vi "Launcher.vi"(8 "error in (no error)":errorcluster, 11 "Launch Local?":bool) -> (0 "error out":errorcluster)   [LabVIEW 2026, in "TALOS.lvlib"]
uses:
  TALOS.lvlib
  Guardian/Guardian/Guardian.lvclass
  C:/LabVIEW Code/TALOS/talos/Ancestor/Ancestor/Ancestor.lvclass
  C:/LabVIEW Code/TALOS/builds/Actor Framework PPL/Actor Framework.lvlibp/1abvi3w/vi.lib/ActorFramework/Actor/Actor.lvclass
  Ancestor/Ancestor/Ancestor.lvclass/Ancestor.ctl
  Support VIs/Global Constants.vi
  Support VIs/Global Memory.vi
  builds/Actor Framework PPL/Actor Framework.lvlibp/1abvi3w/vi.lib/ActorFramework/Actor/Actor.lvclass
  Ancestor/Ancestor/Ancestor.lvclass
panel:
  # "This is just the launcher VI: it only bootstrap the Guardian of this project."
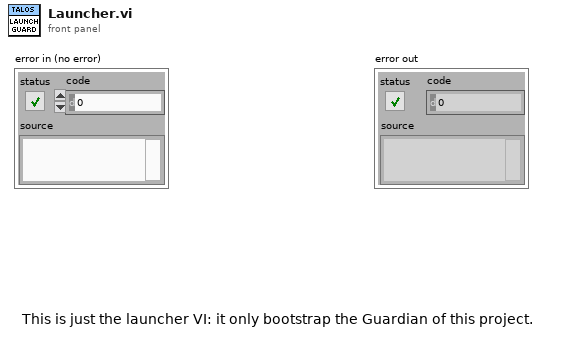
[diagram p1: front panel]
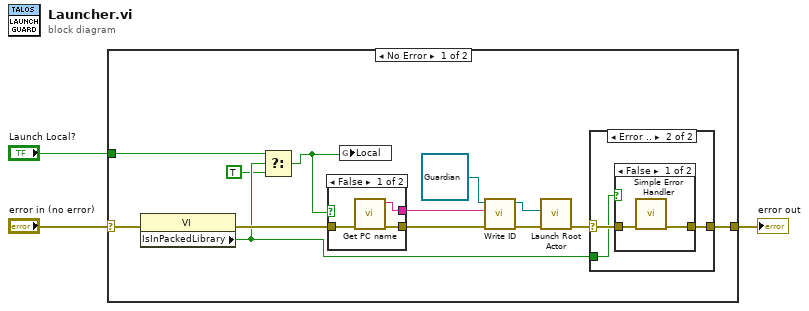
[diagram p0: block diagram]
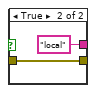
[diagram p4: hidden frame]
diagram:
  n1 = case shown="No Error" "error in (no error)" {
    selector: "error in (no error)" -> [w9 w29]
    tunnel: [w16 w29] -> w3
    tunnel: "Launch Local?" -> [w5 _]
    frame No Error {
      n2 = property class="VI"(error in=w9) -> (error out=w8:errorcluster, "IsInPackedLibrary"=w7:bool)  [unwired: 1 in, 1 out]
      n3 = Select(t=w5, s=w7, f=TRUE) -> (s? t:f=w6:bool)
      n4 = case shown="False" w6 {
        tunnel: w8 -> [w26 w27]
        tunnel: [w25 "local" ("Hostname")] -> w14
        tunnel: [w24 w27] -> w13
        frame False {
          n5 = call "Get PC name.vi"("error in (no error)"=w26) -> ("error out"=w24:errorcluster, "Hostname"=w25:string)  [unwired: 9 in]
        }
        frame True {
        }
      }
      n6 = global write "Global Constants.vi" "Local"(w6) -> ()
      n7 = call "Write ID.vi"("error in (no error)"=w13, "ID"=w14, "Ancestor in"=refnum<class "Guardian.lvclass"> refnum ("Guardian")) -> ("error out"=w10:errorcluster, "Ancestor out"=w11:refnum<class "Guardian.lvclass">)  [unwired: 7 in]
      n8 = call "Launch Root Actor.vi"("error in (no error)"=w10, "Actor"=w11) -> ("error out"=w12:errorcluster)  [unwired: 8 in, 1 out]
      n9 = case shown="Error .." w12 {
        selector: w12 -> [w17 w19]
        tunnel: [w17 w20] -> w16
        tunnel: w7 -> [_ w18]
        frame No Error {
        }
        frame Error {
          n10 = case shown="False" w18 {
            tunnel: [w22 w23] -> w20
            tunnel: w19 -> [w21 w23]
            frame False {
              n11 = call <vilib>:"Simple Error Handler.vi"("error in (no error)"=w21) -> ("error out"=w22:errorcluster)  [unwired: 4 in, 4 out]
            }
            frame True {
            }
          }
        }
      }
    }
    frame Error {
    }
  }
  "error out" <- w3
